vi "MathCad_Matrix_GetRefnum.vi"(3 "error in (no error)":errorcluster, 4 "Variable  Name":string, 5 "Worksheet Reference In":refnum<k7>) -> (0 "error out":errorcluster, 1 "Mathcad.IMatrixValue Refnum":refnum<k7>, 2 "Worksheet Reference Out":refnum<k7>)   [LabVIEW 2015]
doc: "Retrieves a reference from a Mathcad worksheet,based on the variable name. If the variable is defined more than once it is the last value in the worksheet."
panel:
  in  "Mathcad.IMatrixValue Type Descriptor":refnum<k7>
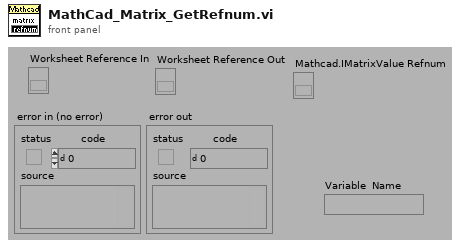
[diagram p1: front panel]
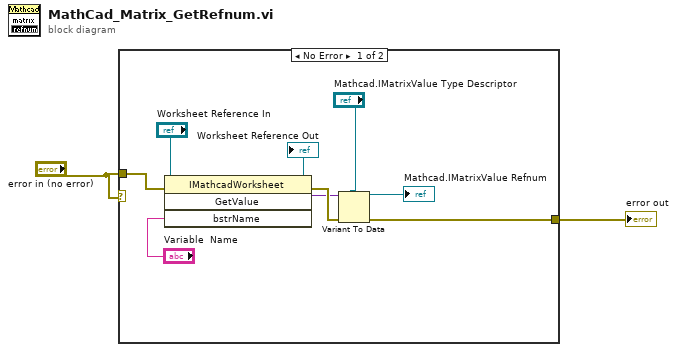
[diagram p0: block diagram]
diagram:
  n1 = case shown="No Error" "error in (no error)" {
    tunnel: [w11 w12] -> w2
    tunnel: "error in (no error)" -> [w5 w12]
    frame No Error {
      n2 = invoke class="IMathcadWorksheet" method="GetValue"(reference="Worksheet Reference In", error in=w5, "bstrName"="Variable  Name") -> (reference out=→"Worksheet Reference Out":refnum<k7>, error out=w8:errorcluster, "GetValue"=w7:variant)  [unwired: 1 in, 1 out]
      n3 = Variant To Data(error in=w8, type="Mathcad.IMatrixValue Type Descriptor", Variant=w7) -> (data=→"Mathcad.IMatrixValue Refnum":refnum<k7>, error out=w11:errorcluster)
    }
    frame Error {
    }
  }
  "error out" <- w2
